vi "Byte Swap Multi-Byte Components.vi"(0 "image pixel data in":u8[](array[numeric]), 5 "data type":T1, 9 "input valid":bool) -> (4 "image pixel data out":u8[](array[numeric]), 10 "output valid":bool)   [LabVIEW 2020, in "GettingStarted_Common_148X_FPGA.lvlib"]
uses:
  GettingStarted_Common_148X_FPGA.lvlib
  <instrlib>/FlexRIO/CSI-2/v2/Common/Types/LLP Data Type.ctl
  <instrlib>/_niInstr/Basic Elements/v1/FPGA/niInstr Basic Elements v1 FPGA.lvlib
  <instrlib>/FlexRIO/CSI-2/v2/Common/NI CSI-2 API Common v2.lvlib
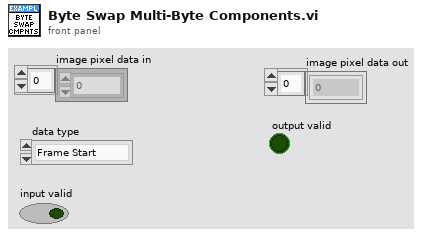
[diagram p1: front panel]
types:
  T1 = typedef "NI CSI-2 API Common v2.lvlib/LLP Data Type.ctl" = enum8{"Frame Start", "Frame End", "Line Start", "Line End", "End of Transmission", "Reserved 0", "Reserved 1", "Reserved 2", "Generic Short Packet 1", "Generic Short Packet 2", "Generic Short Packet 3", "Generic Short Packet 4", "Generic Short Packet 5", "Generic Short Packet 6", "Generic Short Packet 7", "Generic Short Packet 8", "Null", "Blanking Data", "Embedded 8-bit non Image Data", "Generic Long Packet 1", "Generic Long Packet 2", "Generic Long Packet 3", "Generic Long Packet 4", "Reserved 3", "YUV420 8-bit", "YUV420 10-bit", "Legacy YUV420 8-bit", "Reserved 4", "YUV420 8-bit Chroma Shifted", "YUV420 10-bit Chroma Shifted", "YUV422 8-bit", "YUV422 10-bit", "RGB444", "RGB555", "RGB565", "RGB666", "RGB888", "Reserved 5", "Reserved 6", "RAW 24", "RAW 6", "RAW 7", "RAW 8", "RAW 10", "RAW 12", "RAW 14", "RAW 16", "RAW 20", "User Defined 8-bit Data 1", "User Defined 8-bit Data 2", "User Defined 8-bit Data 3", "User Defined 8-bit Data 4", "User Defined 8-bit Data 5", "User Defined 8-bit Data 6", "User Defined 8-bit Data 7", "User Defined 8-bit Data 8", "USL Command", "Reserved 7", "Reserved 8", "Reserved 9", "Reserved 10", "Reserved 11", "Reserved 12", "LRTE EPD Spacer"}
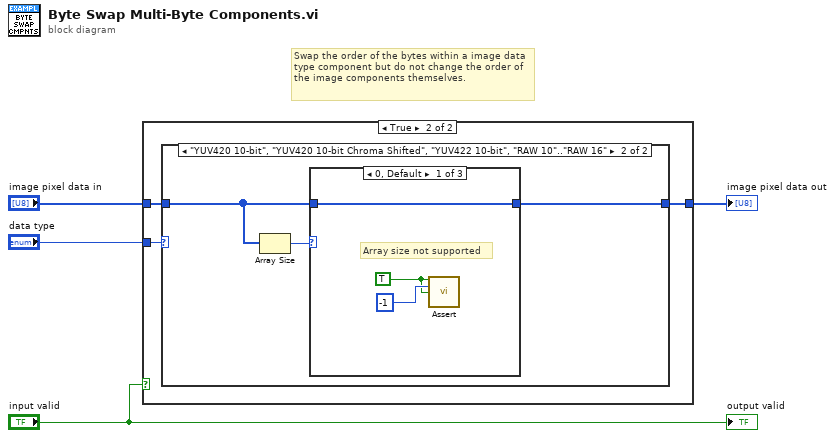
[diagram p0: block diagram]
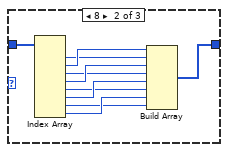
[diagram p4: hidden frame]
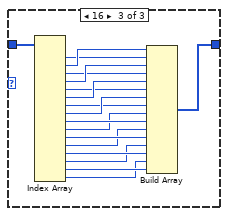
[diagram p5: hidden frame]
diagram:
  # "Swap the order of the bytes within a image data type component but do not change the order of the image components themselves."
  n1 = case shown="True" "input valid" {
    tunnel: "data type" -> [_ w8]
    tunnel: "image pixel data in" -> [w5 w7]
    tunnel: [w5 w6] -> w2
    frame False {
    }
    frame True {
      n2 = case shown="\"YUV420 10-bit\", \"YUV420 10-bit Chroma Shifted\", \"YUV422 10-bit\", \"RAW 10\"..\"RAW 16\"" w8 {
        tunnel: w7 -> [w9 w11]
        tunnel: [w9 w12] -> w6
        frame Default {
        }
        frame "YUV420 10-bit", "YUV420 10-bit Chroma Shifted", "YUV422 10-bit", "RAW 10".."RAW 16" {
          n3 = Array Size(array=w11) -> (size(s)=w10:i32)
          n4 = case shown="0, Default" w10 {
            tunnel: w11 -> [w13 w25 w43]
            tunnel: [w13 w16 w34] -> w12
            frame 0, Default {
              w14 = TRUE ("assert")
              # "Array size not supported"
              n5 = call <instrlib>:"Assert.vi"("assert"=w14, "error code"=-1, "enable show error"=w14) -> ()  [unwired: 13 in]
            }
            frame 8 {
              n6 = Index Array(array=w25) -> (element #1=w20:u8, element #2=w24:u8, element #3=w19:u8, element #4=w23:u8, element #5=w18:u8, element #6=w22:u8, element #7=w17:u8, element #8=w21:u8)  [unwired: 8 in]
              n7 = Build Array(w24, w20, w23, w19, w22, w18, w21, w17) -> (w16:u8[])
            }
            frame 16 {
              n8 = Index Array(array=w43) -> (element #1=w38:u8, element #2=w42:u8, element #3=w37:u8, element #4=w41:u8, element #5=w36:u8, element #6=w40:u8, element #7=w35:u8, element #8=w39:u8, element #9=w30:u8, element #10=w29:u8, element #11=w31:u8, element #12=w28:u8, element #13=w32:u8, element #14=w27:u8, element #15=w33:u8, element #16=w26:u8)  [unwired: 16 in]
              n9 = Build Array(w42, w38, w41, w37, w40, w36, w39, w35, w29, w30, w28, w31, w27, w32, w26, w33) -> (w34:u8[])
            }
          }
        }
      }
    }
  }
  "image pixel data out" <- w2
  "output valid" <- "input valid"
